vi "makeDecisions.vi"(8 "error in (no error)":errorcluster, 10 "model":refnum<class "Model.lvclass">, 11 "MovingToNewForceState in":refnum<class "TransitioningTemperatureState.lvclass">) -> (0 "error out":errorcluster, 2 "model 2":refnum<class "Model.lvclass">, 3 "MovingToNewForceState out":refnum<class "TransitioningTemperatureState.lvclass">)   [LabVIEW 2013, in "TransitioningTemperatureState.lvclass"]
uses:
  TransitioningTemperatureState.lvclass
  Model/Model/Model.lvclass
  MovingToNewTemperatureState/MovingToNewTemperatureState.lvclass
  Typedefs/StateSelector.ctl
  Typedefs/AITDTTypedefs.lvlib
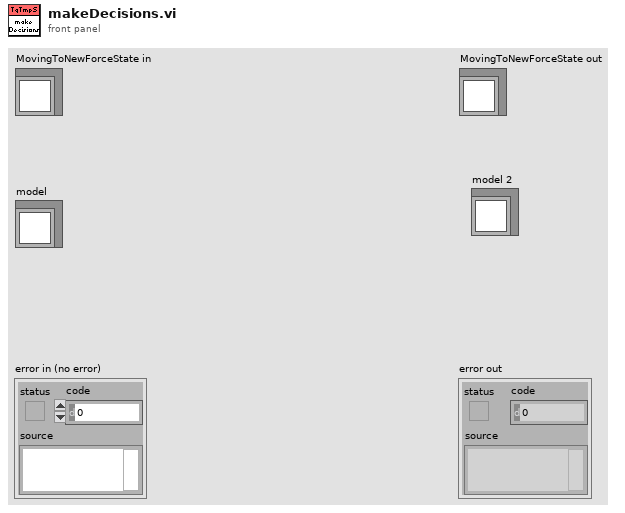
[diagram p1: front panel]
types:
  T1 = typedef "AITDTTypedefs.lvlib/StateSelector.ctl" = enum16{"AwaitingSetpointAcknowledgmentState", "EndingCycleState", "FaultState", "OffState", "PausingState", "RequestingNewSetpointState", "SamplingState", "SettlingState", "SoakingState", "StabilizingState", "StandbyState", "StoppedState", "TransitioningTemperatureState"}
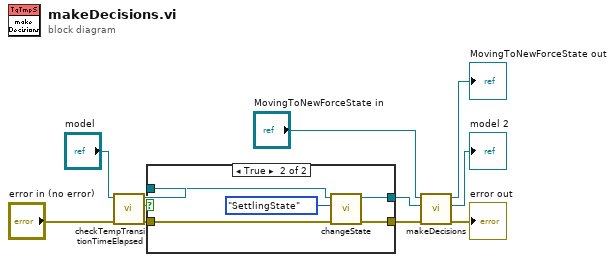
[diagram p0: block diagram]
diagram:
  n1 = call "checkTempTransitionTimeElapsed.vi"("error in (no error)"="error in (no error)", "Model in"="model") -> ("error out"=w3:errorcluster, "tempTransitionTimeHasElapsedIsTrue"=w4:bool, "Model out"=w5:refnum<class "Model.lvclass">)  [unwired: 7 in]
  n2 = case shown="True" w4 {
    tunnel: w5 -> [w13 w18]
    tunnel: w3 -> [w12 w17]
    tunnel: [w13 w15] -> w2
    tunnel: [w12 w14] -> w1
    frame False {
    }
    frame True {
      n3 = call "changeState.vi"("error in (no error)"=w17, "State:"=StateSelector."SettlingState", "Model in"=w18) -> ("error out"=w14:errorcluster, "Model out"=w15:refnum<class "Model.lvclass">)  [unwired: 7 in]
    }
  }
  n4 = call-parent "makeDecisions.vi"("error in (no error)"=w1, "model"=w2, "EnabledState in"="MovingToNewForceState in") -> ("error out"=→"error out":errorcluster, "model 2"=→"model 2":refnum<class "Model.lvclass">, "EnabledState out"=→"MovingToNewForceState out":refnum<class "TransitioningTemperatureState.lvclass">)  [unwired: 6 in]
